vi "flow-builder-delay.vi"(7 "Step Label":string, 11 "Delay [s]":u32) -> (3 "Step Element":T1)   [LabVIEW 2024]
uses:
  controls/UiStepBuilder.ctl
  controls/type.step-builder.ctl
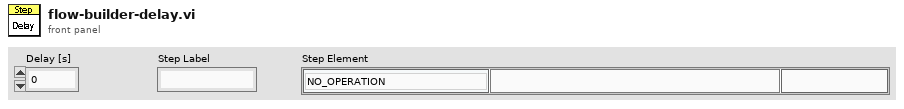
[diagram p1: front panel]
types:
  T1 = typedef "UiStepBuilder.ctl" = cluster{"Step Function":T2, "ParamString":string, "Step Label":string}
  T2 = typedef "type.step-builder.ctl" = enum16{"NO_OPERATION", "DELAY-JUMP", "DELAY", "JUMP", "COMPLETE", "SCHEDULER", "IRR-CHECK", "UNIT-CHECK", "UNIT-SAMPLE", "UNIT-DOSE", "LOG-REPORT", "LOG-MESSAGE", "IO-READ", "IO-READ-MANY", "IO-WRITE", "IO-COMPARE-OUT", "IO-COMPARE-IN", "PROC-START", "PROC-STOP", "PROC-LOAD", "PROC-IS-COMPLETED", "RECORD-MOVE", "GET-RH", "GET-UV", "GET-WD", "GET-WS", "OCS-CHECK", "OCS-RECORD"}
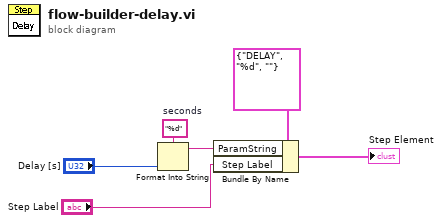
[diagram p0: block diagram]
diagram:
  w5 = "%d"  # seconds
  n1 = Format Into String(format string=w5, "Delay [s]") -> (resulting string=w3:string)  [unwired: 2 in, 1 out]
  n2 = Bundle By Name(cluster=T1 {"Step Function"=enum."DELAY", "ParamString"="%d", "Step Label"=""} ("FlowModeConstant 2"), "ParamString"=w3, "Step Label"="Step Label") -> (→"Step Element":T1)
